vi "Run_Actor_Test.vi"(8 "error in (no error)":errorcluster caption="entrée d'erreur (pas d'erreur)", 11 "Test (Default) en entrée":refnum<class "Actor Test (Default).lvclass">) -> (0 "error out":errorcluster caption="sortie d'erreur", 3 "Test (Default) en sortie":refnum<class "Actor Test (Default).lvclass">)   [LabVIEW 2020, in "Library Core.lvlib" / "Actor Test (Default).lvclass"]
uses:
  Actor Test (Default).lvclass
  Actor Test (Default).lvclass/Actor Test (Default).ctl
  Commun VI/Library Commun.lvlib
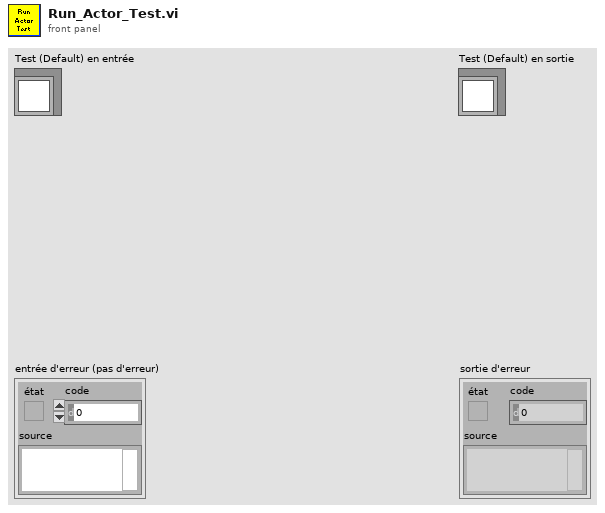
[diagram p1: front panel]
types:
  T1 = enum16{"Get Actor Class", "Set Actor object", "Get Actor object", "List Actor", "Init"}
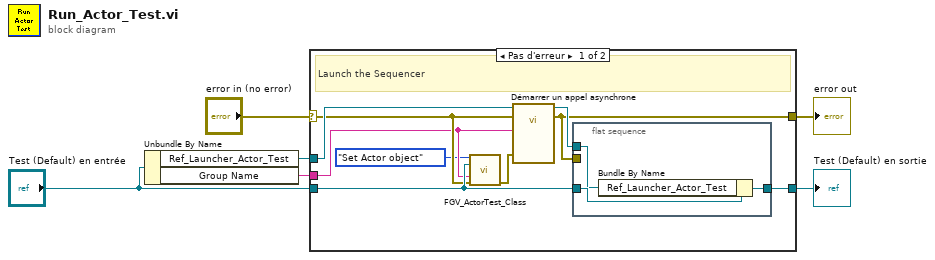
[diagram p0: block diagram]
diagram:
  n1 = Unbundle By Name("Test (Default) en entrée") -> ("Ref_Launcher_Actor_Test"=w6:refnum<vi>, "Group Name"=w2:string)
  n2 = case shown="Pas d'erreur" "error in (no error)" {
    selector: "error in (no error)" -> [w11 w20]
    tunnel: [w7 w20] -> w1
    tunnel: [w15 w19] -> w3
    tunnel: "Test (Default) en entrée" -> [w12 w19]
    tunnel: w6 -> [w14 _]
    tunnel: w2 -> [w9 _]
    frame No Error {
      # "Launch the Sequencer"
      n3 = call "FGV_ActorTest_Class.vi"("Action"=T1."Set Actor object", "Actor Test"=w12, "Group Name"=w9, "error in (no error)"=w11) -> ("error out"=w10:errorcluster)  [unwired: 8 in, 3 out]
      n4 = call-by-ref "Démarrer un appel asynchrone"(reference=w14, error in=w11, 8:"error in (no error)"=w10, "Name Actor"=w9) -> (reference out=w13:refnum<vi>, error out=w7:errorcluster)  [unwired: 6 in, 4 out]
      n5 = flat-sequence {
        tunnel: [w18] -> w15
        tunnel: w12 -> [w17]
        tunnel: w13 -> [w16]
        tunnel: w7 -> [_]
        frame #0 {
          n6 = Bundle By Name(cluster=w17, "Ref_Launcher_Actor_Test"=w16) -> (w18:refnum<class "Actor Test (Default).lvclass">)
        }
      }
    }
    frame Error {
    }
  }
  "error out" <- w1
  "Test (Default) en sortie" <- w3
